vi "LabJackT4_Test_MV.vi"() -> ()   [LabVIEW 2019]
uses:
  sub/enum_dev_id.ctl
  <vilib>/Analysis/baseanly.llb/Mean (DBL).vi
  <vilib>/Analysis/NI_AALBase.lvlib
panel:
  in  "wait_msec":i32=1
  in  "num_read":i32=100
  in  "clear_chart":bool caption="Clear charts to start"
  in  "dev_id":T1
  out "SN":i32
  in  "conn_type":T2(ring)
  out "avg_data":dbl[](array[numeric])
  out "Chart A":waveform(dbl)[](graph)
  out "Last Meas. Time":timestamp format="%<%Y-%m-%d %H:%M:%S>T"
  out "raw_data_size":i32[](array[numeric])
  out "ConnectionType Out":i32
  out "raw_data":dbl[][](array[numeric]) format="%.3f"
  out "Waveform Graph":dbl[][](graph)
  in  "Scan List":string[](array[string])=["AIN0", "AIN1", "AIN2", "AIN3", "AIN4", "AIN5", "AIN6", "AIN7", "AIN8", "AIN9", "AIN10", "AIN11"]
  out "iter":i32
  in  "stop":bool
  out "Error Message":string
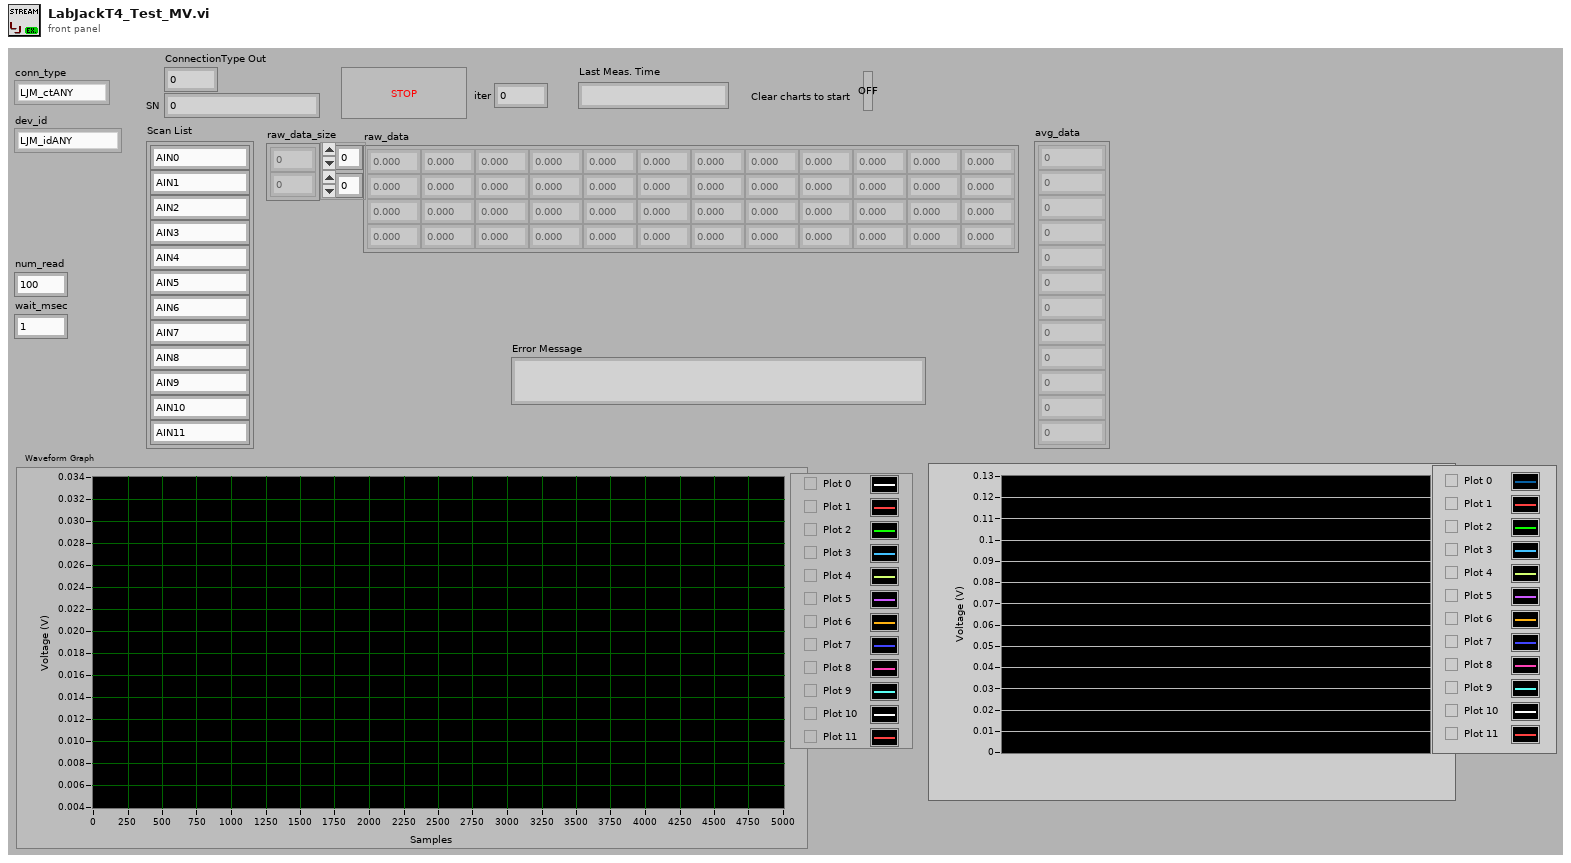
[diagram p1: front panel]
types:
  T1 = typedef "enum_dev_id.ctl" = enum16{"LJM_idANY", "192.168.24.185", "10.0.0.176", "440017305"}
  T2 = enum16{"LJM_ctANY", "LJM_ctUSB", "LJM_ctETHERNET"}
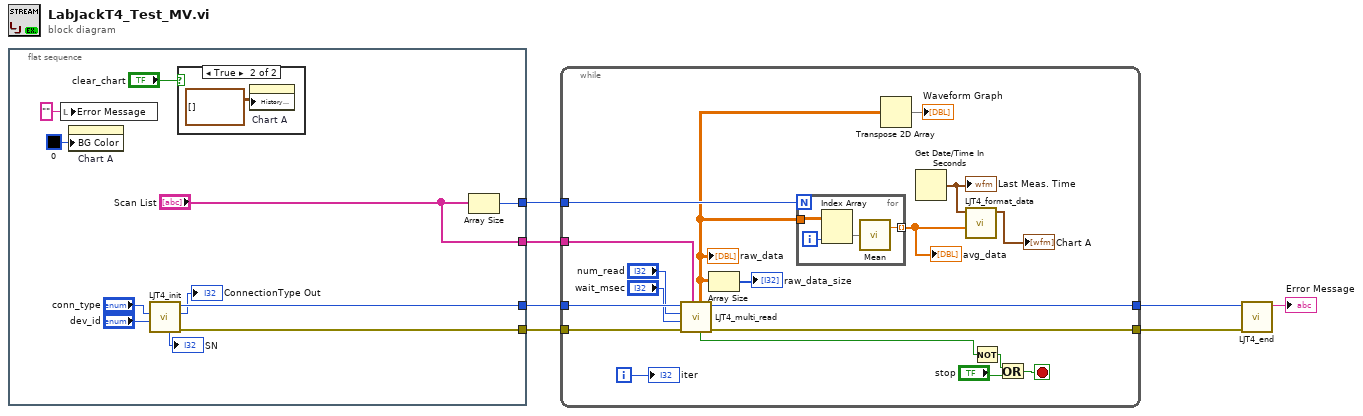
[diagram p0: block diagram]
diagram:
  n1 = flat-sequence {
    tunnel: [w18] -> w7
    tunnel: [w17] -> w6
    tunnel: [w16] -> w2
    tunnel: ["Scan List"] -> w1
    frame #0 {
      n2 = local write "Error Message"("" ("Error Message")) -> ()
      n3 = property on="Chart A" class="WFChart (strict)"("BG Color"=u32 0 ("Plot Area:Colors:BG Color")) -> ()  [unwired: 2 in, 2 out]
      n4 = call "LJT4_init.vi"("dev_id"="dev_id", "conn_type"="conn_type") -> ("error out"=w18:errorcluster, "ConnectionType Out"=→"ConnectionType Out":i32, "Handle Out"=w17:i32, "SN"=→"SN":i32)  [unwired: 5 in, 1 out]
      n5 = case shown="True" "clear_chart" {
        frame False {
        }
        frame True {
          n6 = property on="Chart A" class="WFChart (strict)"("History Data"=waveform(dbl)[][] []) -> ()  [unwired: 2 in, 2 out]
        }
      }
      n7 = Array Size(array="Scan List") -> (size(s)=w16:i32)
    }
  }
  n8 = while {
    tunnel: [w33] -> w4
    tunnel: w6 -> [w34]
    tunnel: w7 -> [w35]
    tunnel: [w32] -> w5
    tunnel: w2 -> [w28]
    tunnel: w1 -> [w23]
    i -> [w36]
    stop <- w37 stop-if-true
    n9 = call "LJT4_multi_read.vi"("aNames"=w23, "error in"=w35, "wait_msec"="wait_msec", "num_read"="num_read", "Handle in"=w34) -> ("error out"=w32:errorcluster, "Handle Out"=w33:i32, "status"=w30:bool, "data_out"=w20:dbl[][])  [unwired: 3 in]
    "raw_data" <- w20
    n10 = Array Size(array=w20) -> (size(s)=→"raw_data_size":i32[])
    n11 = for {
      N: w28 -> [_]
      tunnel: w20 -> [w42]
      tunnel: [w39] -> w27 mode=indexing
      i -> [w41]
      n12 = Index Array(array=w42, index (col)=w41) -> (element=w40:dbl[])  [unwired: 1 in]
      n13 = call-poly <vilib>:"Mean.vi"("X"=w40) -> ("mean"=w39:dbl)  [unwired: 1 out]
    }
    "avg_data" <- w27
    n14 = Transpose 2D Array(2D array=w20) -> (transposed array=→"Waveform Graph":dbl[][])
    n15 = Get Date/Time In Seconds() -> (seconds since 1Jan1904=w26:timestamp)
    "Last Meas. Time" <- w26
    n16 = call "LJT4_format_data.vi"("value_array"=w27, "time"=w26) -> ("waveform_array_A"=→"Chart A":waveform(dbl)[])  [unwired: 9 in]
    n17 = Not(x=w30) -> (.not. x?=w24:bool)
    n18 = Or(x=w24, y="stop") -> (x .or. y?=w37:bool)
    "iter" <- w36
  }
  n19 = call "LJT4_end.vi"("error in (no error)"=w5, "Handle Out"=w4) -> ("String"=→"Error Message":string)  [unwired: 9 in]
